vi "Mask Error.vi"(8 "error in (no error)":errorcluster, 9 "Error Message":string, 10 "Error to Ignore":i32) -> (0 "error out":errorcluster)   [LabVIEW 2019, in "Stanford Research SIM900 Series.lvlib"]
doc: "Mask the speficied execution error number if it occors."
uses:
  Stanford Research SIM900 Series.lvlib
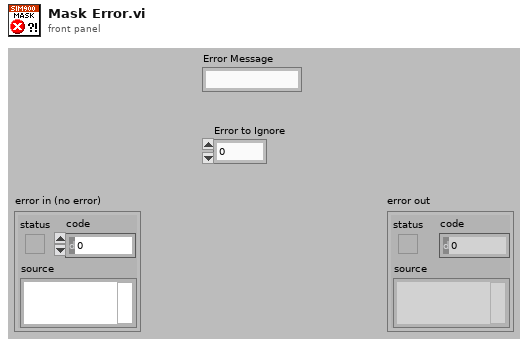
[diagram p1: front panel]
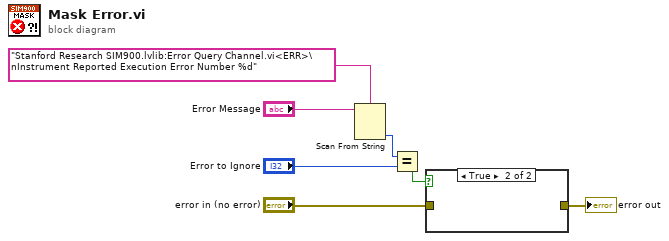
[diagram p0: block diagram]
diagram:
  n1 = Scan From String(format string="Stanford Research SIM900.lvlib:Error Query Channel.vi<ERR>\nInstrument Reported Execution Error Number %d", input string="Error Message") -> (output 1=w6:i32)  [unwired: 3 in, 3 out]
  n2 = Equal?(x=w6, y="Error to Ignore") -> (x = y?=w1:bool)
  n3 = case shown="True" w1 {
    tunnel: "error in (no error)" -> [w8 _]
    tunnel: [w8 _] -> w5
    frame False {
    }
    frame True {
    }
  }
  "error out" <- w5
